vi "dbc-mark-frame.vi"(6 "Value":T1={"Comment"="", "Extended Identifier?"=FALSE, "Transmit Time"=0.0, "Timing Type"=1, "Payload Length"=8, "Identifier"=1, "Frame name"="frame1"} {"Timing Type" items=["Cyclic Data", "Event Data", "Cyclic Remote", "Event Remote"]; "Identifier" format="%010x"}, 7 "tag":string, 8 "error in (no error)":errorcluster, 10 "action":T2, 11 "dbc in":refnum<class "dbc.lvclass">) -> (0 "error out":errorcluster, 3 "dbc out":refnum<class "dbc.lvclass">)   [LabVIEW 2015, in "dbc.lvclass"]
uses:
  dbc.lvclass
  subs/frame.type.ctl
  controls/dbc-frame.ctl
  class.can.table/bAPPdata.lvclass
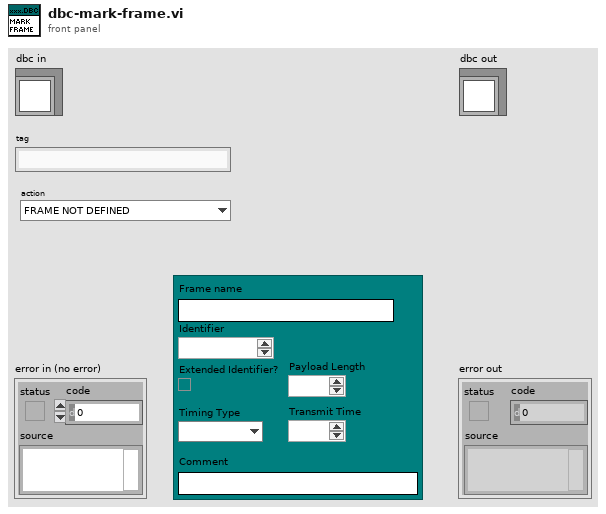
[diagram p1: front panel]
types:
  T1 = typedef "dbc-frame.ctl" = cluster{"Comment":string, "Extended Identifier?":bool, "Transmit Time":dbl, "Timing Type":u32, "Payload Length":u32, "Identifier":u32, "Frame name":string}
  T2 = typedef "frame.type.ctl" = enum16{"FRAME NOT DEFINED", "DUT OUTPUT FRAME", "DUT INPUT FRAME"}
  T3 = typedef "XNET Frame CAN.ctl" = cluster{"timestamp":timestamp, "payload":u8[], "identifier":u32, "type":T4, "extended?":bool, "echo?":bool}
  T4 = typedef "XNET Frame Type CAN.ctl" = u8
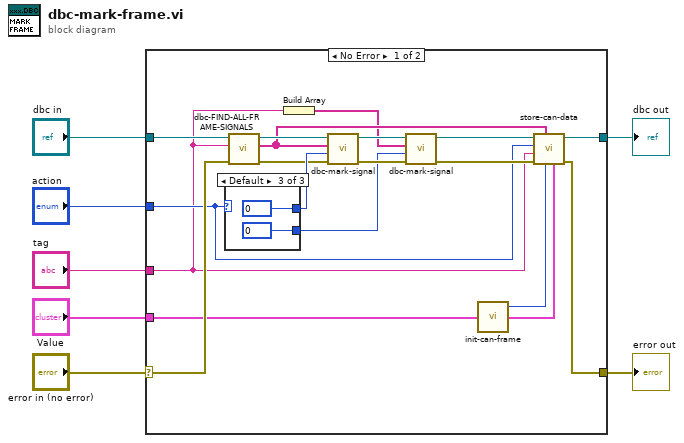
[diagram p0: block diagram]
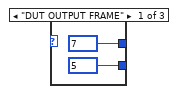
[diagram p2: hidden frame]
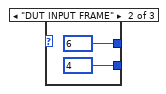
[diagram p3: hidden frame]
diagram:
  n1 = case shown="No Error" "error in (no error)" {
    selector: "error in (no error)" -> [w23 w34]
    tunnel: [w24 w34] -> w6
    tunnel: [w25 w33] -> w4
    tunnel: "dbc in" -> [w26 w33]
    tunnel: "tag" -> [w8 _]
    tunnel: "action" -> [w9 _]
    tunnel: "Value" -> [w22 _]
    frame No Error {
      n2 = case shown="Default" w9 {
        tunnel: [7 6 0] -> w19
        tunnel: [5 4 0] -> w15
        frame "DUT OUTPUT FRAME" {
        }
        frame "DUT INPUT FRAME" {
        }
        frame Default {
        }
      }
      n3 = call "dbc-FIND-ALL-FRAME-SIGNALS.vi"("error in (no error)"=w23, "tag"=w8, "dbc in"=w26) -> ("error out"=w18:errorcluster, "tag.Array"=w14:string[], "dbc out"=w21:refnum<class "dbc.lvclass">)  [unwired: 6 in]
      n4 = Build Array(w8) -> (w13:string[])
      n5 = call "dbc-mark-signal.vi"("error in (no error)"=w18, "Numeric"=w19, "Array"=w14, "dbc in"=w21) -> ("error out"=w16:errorcluster, "dbc out"=w20:refnum<class "dbc.lvclass">)  [unwired: 6 in]
      n6 = call "dbc-mark-signal.vi"("error in (no error)"=w16, "Numeric"=w15, "Array"=w13, "dbc in"=w20) -> ("error out"=w12:errorcluster, "dbc out"=w17:refnum<class "dbc.lvclass">)  [unwired: 6 in]
      n7 = call "init-can-frame.vi"("selected.frame"=w22) -> ("CAN frame"=w11:T3, "Identifier"=w10:u32)  [unwired: 3 in]
      n8 = call "store-can-data.vi"("CAN frame"=w11, "id"=w10, "child.tags"=w14, "error in (no error)"=w12, "tag"=w8, "frame.type"=w9, "CANtable in"=w17) -> ("error out"=w24:errorcluster, "CANtable out"=w25:refnum<class "dbc.lvclass">)  [unwired: 3 in]
    }
    frame Error {
    }
  }
  "error out" <- w6
  "dbc out" <- w4
